vi "SignalGenerator.vi"(1 "Stop":bool, 2 "Amplitude":dbl=1.0, 3 "Frequency":dbl=10.1) -> (0 "error out":errorcluster)   [LabVIEW 2015]
panel:
  out "error in (no error)":errorcluster
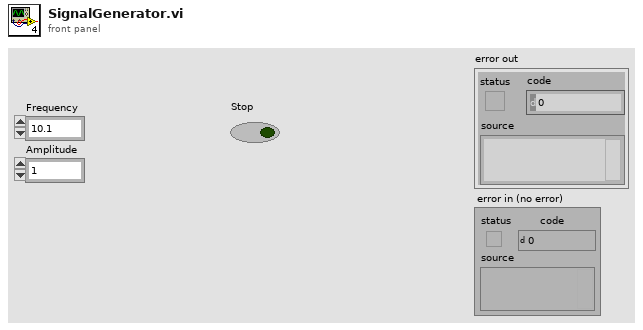
[diagram p1: front panel]
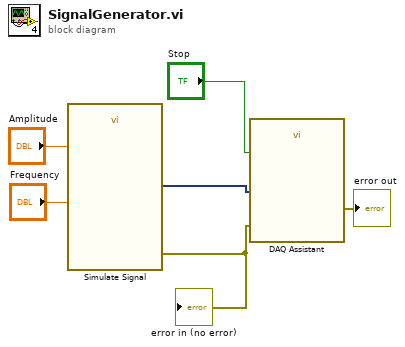
[diagram p0: block diagram]
diagram:
  n1 = call "Simulate Signal"("Frequency"="Frequency", "Amplitude"="Amplitude") -> ("Sine"=w6:dynamicdata, "error out"=w2:errorcluster)  [unwired: 12 in]
  "error in (no error)" <- w2
  n2 = call "DAQ Assistant"("data"=w6, "error in"=w2, "stop (F)"="Stop") -> ("error out"=→"error out":errorcluster)  [unwired: 14 in, 2 out]
